vi "Pockels Cal-Cal range entry window.vi"(11 "Calibration data array (inc. data header row)":string[][](array[string])=[["Pockels V", "No objective"], ["0.0", "0"], ["0.1", "11.0"], ["0.2", "56"], ["0.3", "80"], ["0.4", "90"], ["0.5", "95"], ["0.6", "110"], ["0.7", "140"], ["0.8", "150"], ["0.9", "170"], ["1.0", "190"], ["1.1", "200"], ["1.2", "212"], ["1.3", "219"], ["1.4", "235"], ["1.5", "245"], ["1.6", "251"], ["1.7", "248"], ["1.8", "240"], ["1.9", "230"], ["2.0", "225"]]) -> (1 "Cancelled":bool, 3 "Cal subset info array":string[][](array[string]))   [LabVIEW 2020]
uses:
  <vilib>/Utility/miscctls.llb/LVPointTypeDef.ctl
  Typedefs/Pockels cal processing type.ctl
  Globals/gl_Calibration globals.vi
  Global Variables/General Globals.vi
panel:
  in  "Close":bool
  in  "Use cal subset":bool
  out "Instructions":string="  Using the two red vertical cursors you may specify just the useful section to be used.\n  Place one cursor at the pockels voltage resulting in the minimum power. Place the other cursor at the desired maximum.\n  The black curve named \"No Objective\" is the actual calibration curve used by the microscope software.\n  The rest of the curves are present for informational purposes only."
  in  "Cancel":bool
  in  "Pockels Calibration Graph":cluster{cluster{"Value":dbl, "Value":dbl}[]}[](graph)
  in  "Use whole cal":bool
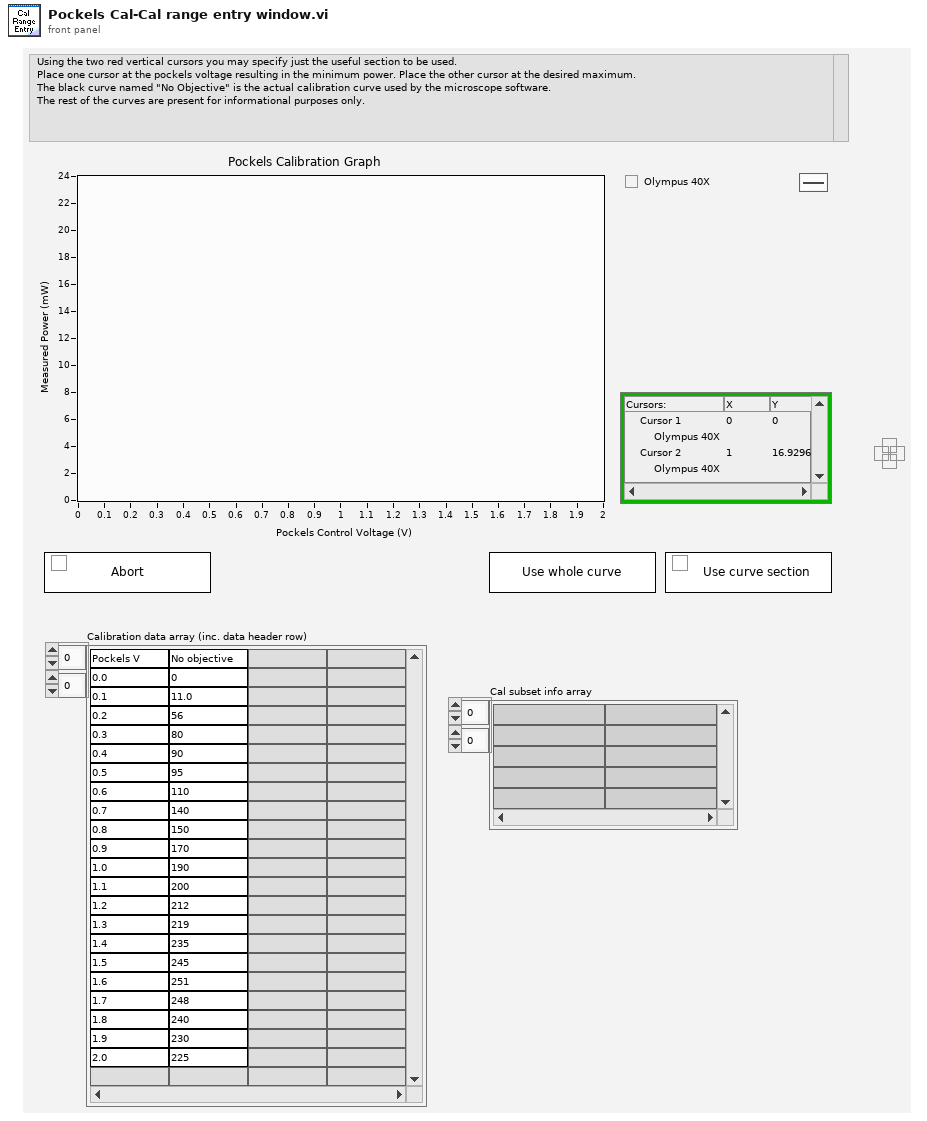
[diagram p1: front panel]
types:
  T1 = typedef "Pockels cal processing type.ctl" = enum16{"Interpolate", "Condense"}
  T2 = enum16{"Set cursors dynamically", "Set cursors from file"}
  T3 = typedef "LVPointTypeDef.ctl" = cluster{"Horizontal":i16, "Vertical":i16}
  T4 = cluster{"This VI":refnum<vi>, "Pockels Calibration Graph":refnum<vi>, "Instructions":refnum<vi>, "Close":refnum<vi>, "Use cal subset":refnum<vi>, "Use whole cal":refnum<vi>}
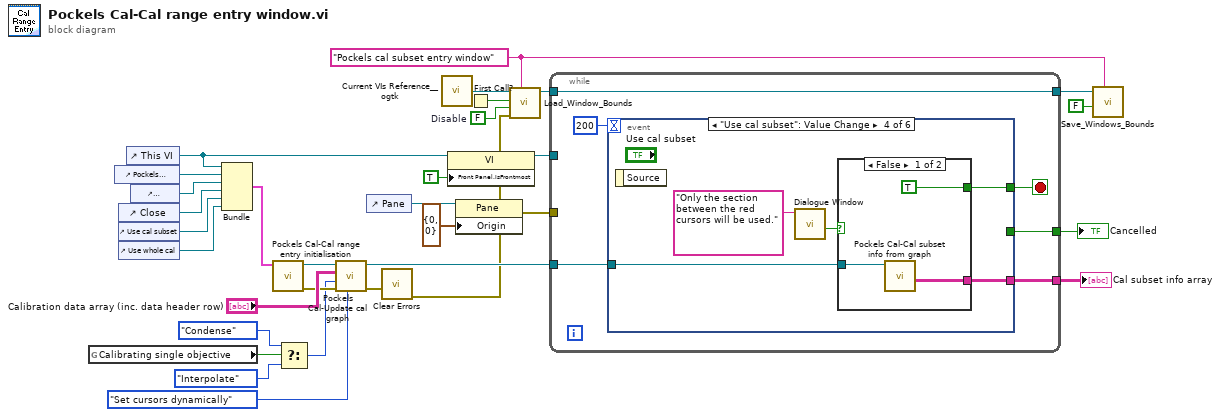
[diagram p0: block diagram]
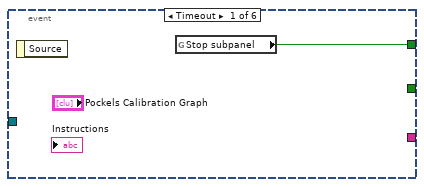
[diagram p2: hidden frame]
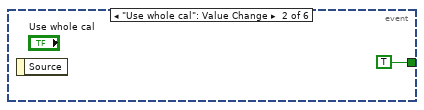
[diagram p3: hidden frame]
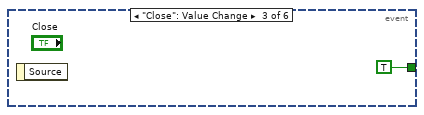
[diagram p4: hidden frame]
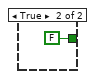
[diagram p5: hidden frame]
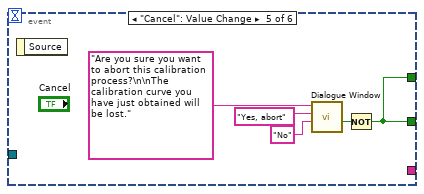
[diagram p6: hidden frame]
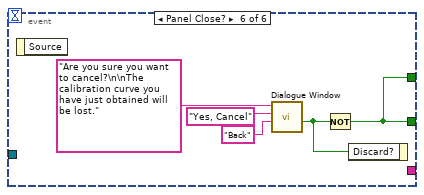
[diagram p7: hidden frame]
diagram:
  w26 = FALSE  # Disable
  w25 = "Pockels cal subset entry window" ("Window Name (i.e. Key)")
  n1 = global read "gl_Calibration globals.vi" "Calibrating single objective"() -> (w15:bool)
  n2 = control-ref of="Pockels Calibration Graph"() -> (w6:refnum<vi>)
  n3 = control-ref of="Close"() -> (w4:refnum<vi>)
  n4 = control-ref of="Use cal subset"() -> (w3:refnum<vi>)
  n5 = control-ref of="Use whole cal"() -> (w2:refnum<vi>)
  n6 = control-ref of="This VI"() -> (w7:refnum<vi>)
  n7 = control-ref of="Instructions"() -> (w5:refnum<vi>)
  n8 = Bundle("This VI"=w7, "Pockels Calibration Graph"=w6, "Instructions"=w5, "Close"=w4, "Use cal subset"=w3, "Use whole cal"=w2) -> (w1:T4)  [unwired: 1 in]
  n9 = call "Pockels Cal-Cal range entry initialisation.vi"("Cluster"=w1) -> ("error out"=w13:errorcluster, "XYGraph out"=w10:refnum<vi>)  [unwired: 9 in]
  n10 = Select(t=Pockels_cal_processing_type."Condense" ("Processing Type (Interpolate)"), s=w15, f=Pockels_cal_processing_type."Interpolate" ("Processing Type (Interpolate)")) -> (s? t:f=w8:T1)
  n11 = call "Pockels Cal-Update cal graph.vi"("Function"=T2."Set cursors dynamically", "error in (no error)"=w13, "Processing Type (Interpolate)"=w8, "Cal table"="Calibration data array (inc. data header row)", "XYGraph in"=w10) -> ("error out"=w12:errorcluster, "XYGraph"=w20:refnum<vi>)  [unwired: 5 in]
  n12 = control-ref of="Pane"() -> (w21:refnum<vi>)
  n13 = call <vilib>:"Clear Errors.vi"("error in (no error)"=w12) -> ("error out"=w11:errorcluster)  [unwired: 5 in, 1 out]
  n14 = call <userlib>:"Current VIs Reference__ogtk.vi"() -> ("Current VI's reference"=w28:refnum<vi>)  [unwired: 5 in]
  n15 = property on="Property Node" class="VI"(reference=w7, "Front Panel.IsFrontmost"=TRUE ("Front Panel Window:Is Frontmost")) -> (reference out=w31:refnum<vi>)  [unwired: 1 in, 1 out]
  n16 = property class="Pane"(reference=w21, "Origin"=T3 {"Horizontal"=0, "Vertical"=0}) -> (error out=w29:errorcluster)  [unwired: 1 in, 1 out]
  n17 = First Call?() -> (First Call?: T/F=w27:bool)
  n18 = call "Load_Window_Bounds.vi"("Window Name (i.e. Key)"=w25, "error in"=w11, "Disable"=w26, "First Call"=w27, "Window VI's Ref"=w28) -> ("reference out"=w23:refnum<vi>)  [unwired: 3 in, 3 out]
  n19 = while {
    tunnel: w29 -> [_]
    tunnel: w31 -> [_]
    tunnel: w23 -> [w36]
    tunnel: [w36] -> w22
    tunnel: w20 -> [w35]
    tunnel: [w34] -> w16
    tunnel: [w33] -> w18
    stop <- w38 stop-if-true
    n20 = event shown="[3] \"Use cal subset\": Value Change" {
      selector: _ -> [_ _ _ _ _ _]
      dyn-events: _ -> [_ _ _ _ _ _]
      timeout: 200 -> [_ _ _ _ _ _]
      tunnel: [w39 TRUE ("Stop?") TRUE ("Stop?") w46 w51 w57] -> w38
      tunnel: w35 -> [_ _ _ w45 _ _]
      tunnel: [_ _ _ w44 _ _] -> w34
      tunnel: [_ _ _ _ w51 w57] -> w33
      event Timeout {
        n21 = event-data() -> ()  [unwired: 1 in, 1 out]
        n22 = global read "General Globals.vi" "Stop subpanel"() -> (w39:bool)
      }
      event "Use whole cal": Value Change {
        n23 = event-data() -> ()  [unwired: 1 in, 1 out]
      }
      event "Close": Value Change {
        n24 = event-data() -> ()  [unwired: 1 in, 1 out]
      }
      event "Use cal subset": Value Change {
        n25 = event-data() -> ()  [unwired: 1 in, 1 out]
        n26 = call "Dialogue Window.vi"("Message string"="Only the section between the red cursors will be used.") -> ("Cancelled (Left button pressed)"=w43:bool)  [unwired: 8 in, 2 out]
        n27 = case shown="False" w43 {
          tunnel: [TRUE ("Stop?") FALSE ("Stop?")] -> w46
          tunnel: w45 -> [w48 _]
          tunnel: [w47 _] -> w44
          frame False {
            n28 = call "Pockels Cal-Cal subset info from graph.vi"("XYGraph in"=w48) -> ("Cal subset info array"=w47:string[][])  [unwired: 8 in, 2 out]
          }
          frame True {
          }
        }
      }
      event "Cancel": Value Change {
        n29 = event-data() -> ()  [unwired: 1 in, 1 out]
        n30 = call "Dialogue Window.vi"("Caption-Left button (Cancel)"="No" ("Caption-Right button (OK)"), "Caption-Right button (OK)"="Yes, abort" ("Caption-Left button (Cancel)"), "Message string"="Are you sure you want to abort this calibration process?\n\nThe calibration curve you have just obtained will be lost.") -> ("Cancelled (Left button pressed)"=w52:bool)  [unwired: 6 in, 2 out]
        n31 = Not(x=w52) -> (.not. x?=w51:bool)
      }
      event Panel Close? {
        n32 = event-data() -> ()  [unwired: 1 in, 1 out]
        n33 = call "Dialogue Window.vi"("Caption-Left button (Cancel)"="Back" ("Caption-Right button (OK)"), "Caption-Right button (OK)"="Yes, Cancel" ("Caption-Left button (Cancel)"), "Message string"="Are you sure you want to cancel?\n\nThe calibration curve you have just obtained will be lost.") -> ("Cancelled (Left button pressed)"=w56:bool)  [unwired: 6 in, 2 out]
        n34 = Not(x=w56) -> (.not. x?=w57:bool)
        n35 = event-data("Discard?"=w56) -> ()  [unwired: 1 in, 1 out]
      }
    }
  }
  "Cancelled" <- w18
  "Cal subset info array" <- w16
  n36 = call "Save_Windows_Bounds.vi"("Window Name (i.e. Key)"=w25, "Front Panel Window:Open"=FALSE, "Window VI's Ref"=w22) -> ()  [unwired: 8 in, 1 out]
